vi "SSC DCPower Filter Pins.vi"(0 "DCPower SSC in":T1[](array[typedef]), 5 "Requested Pins":tag[](array[tag]), 11 "error in":errorcluster) -> (4 "Filtered DCPower SSC out":T1[](array[typedef]), 15 "error out":errorcluster)   [LabVIEW 2020]
doc: "This VI filters the TSM SSC cluster to requested pins."
uses:
  SSC DCPower/SSC DCPower.ctl
  Shared SubVIs/Trim Whitespace [Inlined].vi
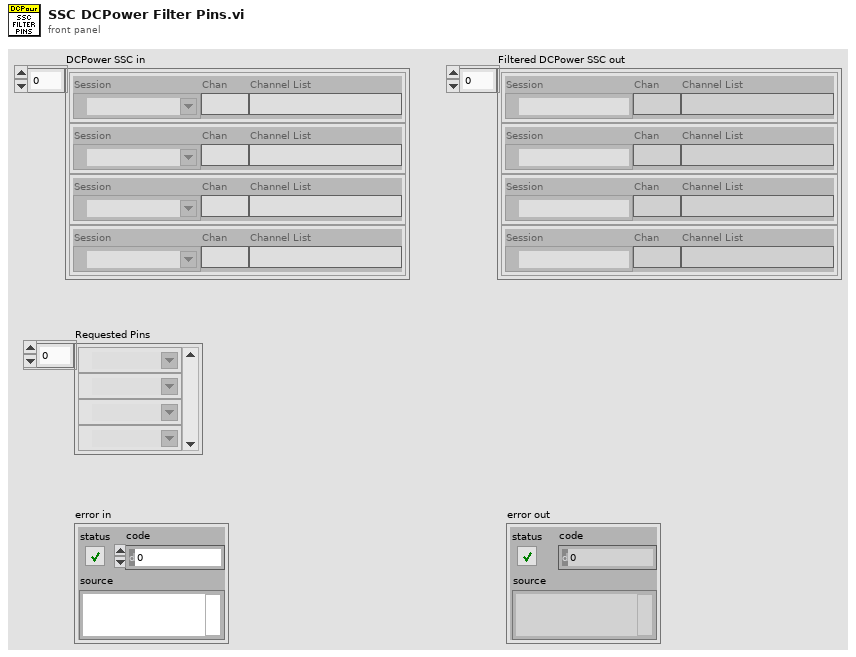
[diagram p1: front panel]
types:
  T1 = typedef "SSC DCPower.ctl" = cluster{"Session":refnum<k15>, "Chan":string, "Channel List":string}
  T2 = cluster{"trimmed string":i32, "index of element":i32, "DCPower SSC in":T1}
  T3 = cluster{"trimmed string":i32, "index of element":i32, "DCPower SSC in":T1}[]
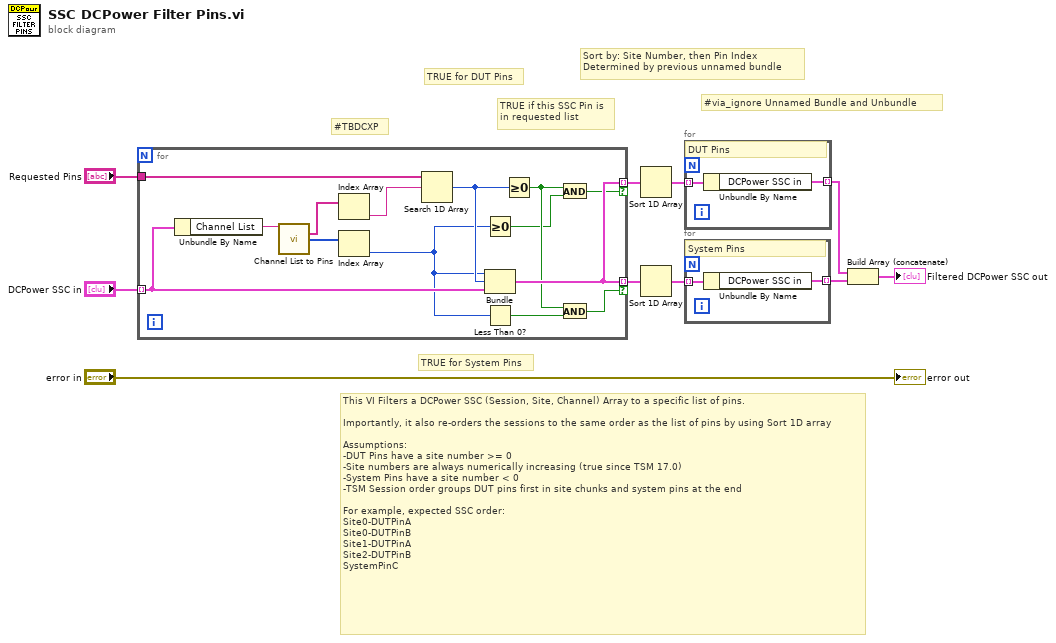
[diagram p0: block diagram]
diagram:
  # "#TBDCXP"
  # "#via_ignore Unnamed Bundle and Unbundle"
  # "TRUE for DUT Pins"
  # "TRUE for System Pins"
  # "TRUE if this SSC Pin is\nin requested list"
  # "Sort by: Site Number, then Pin Index\nDetermined by previous unnamed bundle"
  # "This VI Filters a DCPower SSC (Session, Site, Channel) Array to a specific list of pins.\n\nImportantly, it also re-orders the sessions to the same order as the list of pins by using Sort 1D array\n\nAssumptions:\n-DUT Pins have a site number >= 0\n-Site numbers are always numerically increasing (true since TSM 17.0)\n-System Pins have a site number < 0\n-TSM Session order groups DUT pins first in site chunks and system pins at the end\n\nFor example, expected SSC order:\nSite0-DUTPinA\nSite0-DUTPinB\nSite1-DUTPinA\nSite2-DUTPinB\nSystemPinC"
  n1 = for {
    tunnel: "Requested Pins" -> [w24]
    tunnel: "DCPower SSC in" -> [w16] mode=indexing
    tunnel: [w22] -> w6 mode=indexing if=w20
    tunnel: [w22] -> w7 mode=indexing if=w21
    n2 = Unbundle By Name(w16) -> ("Channel List"=w15:string)
    n3 = call "Channel List to Pins.vi"("Channel List"=w15) -> ("Pins"=w14:tag[], "Sites"=w12:i32[])  [unwired: 12 in, 1 out]
    n4 = Index Array(array=w14) -> (element=w13:tag)  [unwired: 1 in]
    n5 = Index Array(array=w12) -> (element=w11:i32)  [unwired: 1 in]
    n6 = Search 1D Array(1D array=w24, element=w13) -> (index of element=w23:i32)  [unwired: 1 in]
    n7 = Greater Or Equal To 0?(x=w11) -> (x >= 0?=w17:bool)
    n8 = Bundle("trimmed string"=w11, "index of element"=w23, "DCPower SSC in"=w16) -> (w22:T2)  [unwired: 1 in]
    n9 = Less Than 0?(x=w11) -> (x < 0?=w18:bool)
    n10 = Greater Or Equal To 0?(x=w23) -> (x >= 0?=w19:bool)
    n11 = And(x=w19, y=w17) -> (x .and. y?=w21:bool)
    n12 = And(x=w19, y=w18) -> (x .and. y?=w20:bool)
  }
  n13 = Sort 1D Array(array=w7) -> (sorted array=w5:T3)
  n14 = Sort 1D Array(array=w6) -> (sorted array=w4:T3)
  n15 = for {
    tunnel: w5 -> [w26] mode=indexing
    tunnel: [w25] -> w3 mode=indexing
    # "DUT Pins"
    n16 = Unbundle By Name(w26) -> ("DCPower SSC in"=w25:T1)
  }
  n17 = for {
    tunnel: w4 -> [w28] mode=indexing
    tunnel: [w27] -> w2 mode=indexing
    # "System Pins"
    n18 = Unbundle By Name(w28) -> ("DCPower SSC in"=w27:T1)
  }
  n19 = Build Array (concatenate)(w3, w2) -> (→"Filtered DCPower SSC out":T1[])
  "error out" <- "error in"
